vi "Hash.vi"(8 "error in (no error)":errorcluster, 10 "Message":string, 11 "SHA-1 in":refnum<class "SHA-1.lvclass">) -> (0 "error out":errorcluster, 2 "Hash":string, 3 "SHA-1 out":refnum<class "SHA-1.lvclass">)   [LabVIEW 2020, in "Crypto.lvlib" / "SHA-1.lvclass"]
uses:
  SHA-1.lvclass
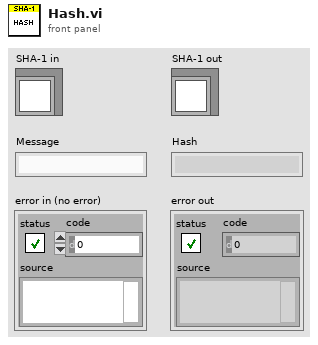
[diagram p1: front panel]
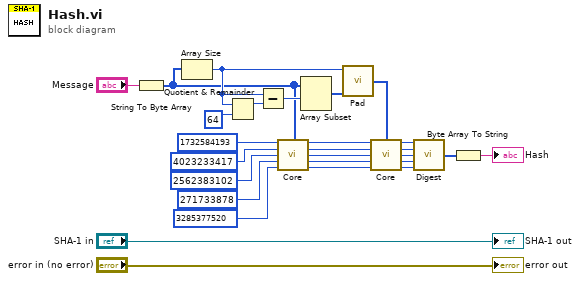
[diagram p0: block diagram]
diagram:
  n1 = String To Byte Array(string="Message") -> (unsigned byte array=w8:u8[])
  n2 = Array Size(array=w8) -> (size(s)=w10:i32)
  n3 = Quotient & Remainder(x=w10, y=64) -> (x-y*floor(x/y)=w13:i32)  [unwired: 1 out]
  n4 = Subtract(x=w10, y=w13) -> (x-y=w14:i32)
  n5 = call "Core.vi"("s1"=u32 1732584193, "Input Bytes"=w8, "s2"=u32 4023233417, "s3"=u32 2562383102, "s4"=u32 271733878, "s5"=u32 3285377520 ("s4")) -> ("s1 out"=w20:u32, "s2 out"=w19:u32, "s3 out"=w18:u32, "s4 out"=w17:u32, "s5 out"=w16:u32)  [unwired: 5 in]
  n6 = Array Subset(array=w8, index=w14) -> (w11:u8[])  [unwired: 1 in]
  n7 = call "Pad.vi"("Message Length (bytes)"=w10, "Last Part"=w11) -> ("Padding"=w15:u8[])  [unwired: 13 in]
  n8 = call "Core.vi"("s1"=w20, "Input Bytes"=w15, "s2"=w19, "s3"=w18, "s4"=w17, "s5"=w16) -> ("s1 out"=w7:u32, "s2 out"=w6:u32, "s3 out"=w5:u32, "s4 out"=w4:u32, "s5 out"=w3:u32)  [unwired: 5 in]
  n9 = call "Digest.vi"("s1"=w7, "s2"=w6, "s3"=w5, "s4"=w4, "s5"=w3) -> ("message-digest"=w2:u8[])  [unwired: 10 in]
  n10 = Byte Array To String(unsigned byte array=w2) -> (string=→"Hash":string)
  "error out" <- "error in (no error)"
  "SHA-1 out" <- "SHA-1 in"
